vi "GetClass.vi"(8 "error in (no error)":errorcluster, 11 "NI Card in":refnum<class "NI Card.lvclass">) -> (0 "error out":errorcluster, 2 "Device Class":string="NI Card", 3 "NI Card out":refnum<class "NI Card.lvclass">)   [LabVIEW 2013, in "NI Card.lvclass"]
uses:
  NI Card.lvclass
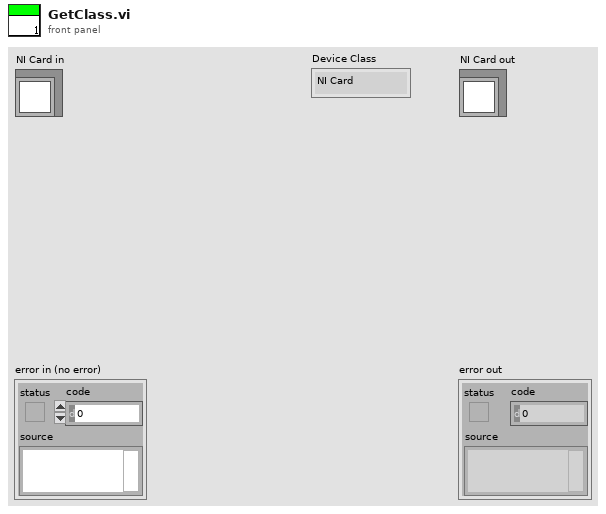
[diagram p1: front panel]
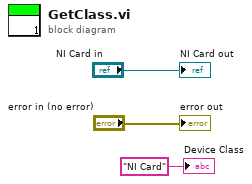
[diagram p0: block diagram]
diagram:
  "error out" <- "error in (no error)"
  "NI Card out" <- "NI Card in"
  "Device Class" <- "NI Card"
